vi "get encoder settings.vi"(8 "error in (no error)":errorcluster, 10 "encoder_settings":T1, 11 "id":i32) -> (0 "error out":errorcluster, 2 "encoder_settings out":T1, 3 "function return":i32)   [LabVIEW 2012, in "libximc.lvlib"]
doc: "result_t XIMC_API get_encoder_settings (device_t id, encoder_settings_t* encoder_settings);"
uses:
  libximc.lvlib
  libximc.dll
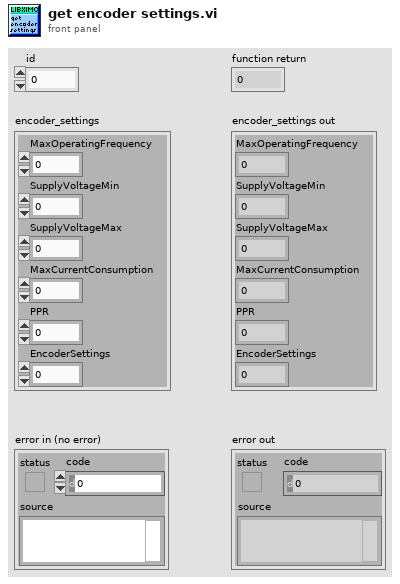
[diagram p1: front panel]
types:
  T1 = cluster{"MaxOperatingFrequency":sgl, "SupplyVoltageMin":sgl, "SupplyVoltageMax":sgl, "MaxCurrentConsumption":sgl, "PPR":u32, "EncoderSettings":u32}
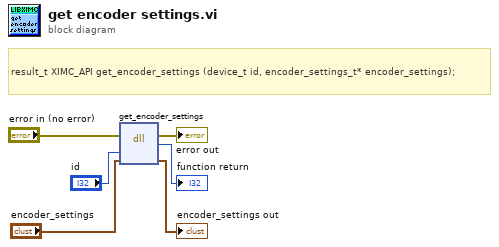
[diagram p0: block diagram]
diagram:
  # "result_t XIMC_API get_encoder_settings (device_t id, encoder_settings_t* encoder_settings);"
  n1 = dll-call lib="C:/Users/Stepan/Downloads/labview_2.9.11_testgen_thread/libximc.*" fn="get_encoder_settings"(error in="error in (no error)", "id"="id", "encoder_settings"="encoder_settings") -> (error out=→"error out":errorcluster, →"function return":i32, "encoder_settings"=→"encoder_settings out":T1)  [unwired: 3 in, 1 out]
